vi "VI Server_Set Signaling Value of Menu Ring by Item Selection.vi"(6 "Item":string, 7 "Label":string, 8 "error in (no error)":errorcluster, 11 "VI Server Cluster.DUP in":T1) -> (0 "error out":errorcluster, 3 "VI Server Cluster.DUP out":T1)   [LabVIEW 2020]
uses:
  VI Server_TypeDefs/VI Server_RefsCluster.ctl
  VI Server Toolkit LV2013.lvlib
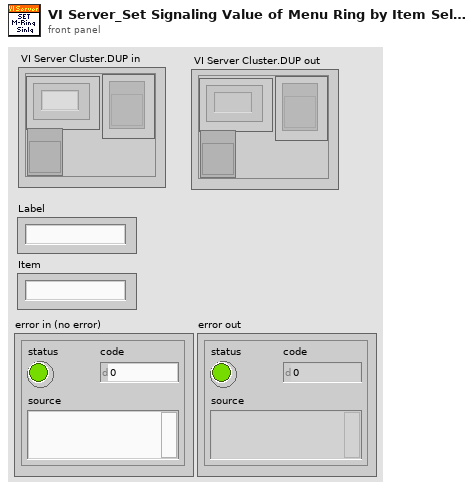
[diagram p1: front panel]
types:
  T1 = typedef "VI Server_RefsCluster.ctl" = cluster{"Labels":string[], "Refs":refnum<vi>[], "VI Ref":refnum<vi>}
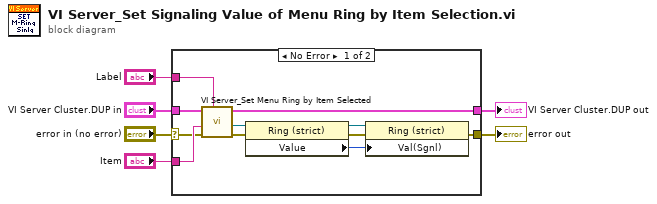
[diagram p0: block diagram]
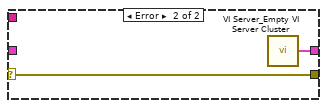
[diagram p2: hidden frame]
diagram:
  n1 = case shown="No Error" "error in (no error)" {
    selector: "error in (no error)" -> [w7 w19]
    tunnel: [w15 w19] -> w6
    tunnel: "VI Server Cluster.DUP in" -> [w11 _]
    tunnel: "Item" -> [w10 _]
    tunnel: "Label" -> [w9 _]
    tunnel: [w8 w18] -> w2
    frame No Error {
      n2 = call "VI Server_Set Menu Ring by Item Selected.vi"("Label"=w9, "error in"=w7, "Item"=w10, "VI Server Cluster"=w11) -> ("error out"=w12:errorcluster, "Control Reference"=w13:refnum<vi>, "VI Server Cluster.DUP"=w8:T1)  [unwired: 5 in]
      n3 = property class="Ring (strict)"(reference=w13, error in=w12) -> (reference out=w16:refnum<vi>, error out=w14:errorcluster, "Value"=w17:u16)
      n4 = property class="Ring (strict)"(reference=w16, error in=w14, "Val(Sgnl)"=w17) -> (error out=w15:errorcluster)  [unwired: 1 out]
    }
    frame Error {
      n5 = call "VI Server_Empty VI Server Cluster.vi"() -> ("VI Server Cluster"=w18:T1)  [unwired: 7 in]
    }
  }
  "error out" <- w6
  "VI Server Cluster.DUP out" <- w2
